vi "External Time to System Time.vi"(8 "error in (no error)":errorcluster, 9 "ClockID":u8, 10 "External Time":i64, 11 "Clock Convert Map in":T1) -> (0 "error out":errorcluster, 1 "Last Reset Time":u64, 2 "System Time":i64, 3 "Clock Convert Map out":T1)   [LabVIEW 2021, in "CIFClocks.lvlib"]
uses:
  CIFClocks.lvlib
  Typedef/Clock Conversion Map.ctl
  Typedef/Timestamp Pair.ctl
  CIFCore/Common/Typedef/Errors.ctl
  CIFCore/Common/Utilities/Append Error Location.vi
  CIFCore/Common/CIFCoreCommon.lvlib
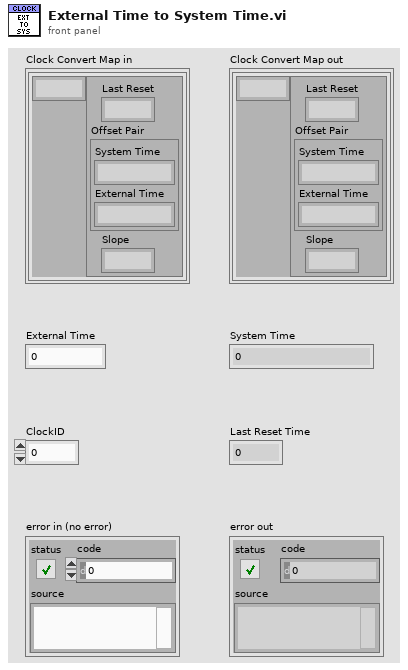
[diagram p1: front panel]
types:
  T1 = typedef "CIFClocks.lvlib/Clock Conversion Map.ctl" = map{u8, cluster{"Last Reset":u64, "Offset Pair":T2, "Slope":dbl}}
  T2 = typedef "CIFClocks.lvlib/Timestamp Pair.ctl" = cluster{"System Time":i64, "External Time":i64}
  T3 = cluster{"Last Reset":u64, "Offset Pair":T2, "Slope":dbl}
  T4 = typedef "CIFCoreCommon.lvlib/Errors.ctl" = enum16{"Invalid Clock ID", "Long Sleep", "gRPC Server Not Found", "Config Parse", "Timestamp Wrap", "Delayed Execution", "Duplicate Channel", "Missing Channel", "Incorrect Type", "Flatten Error", "Unflatten Data", "Unique Name", "Plugin Not Found", "Plugin Type Not Found", "Plugin Version Not Found", "Manager Not Found", "Numerical Issue", "Time Jump", "Clock ID Match", "Channel Length", "Plugin Connection", "gRPC Server Connection"}
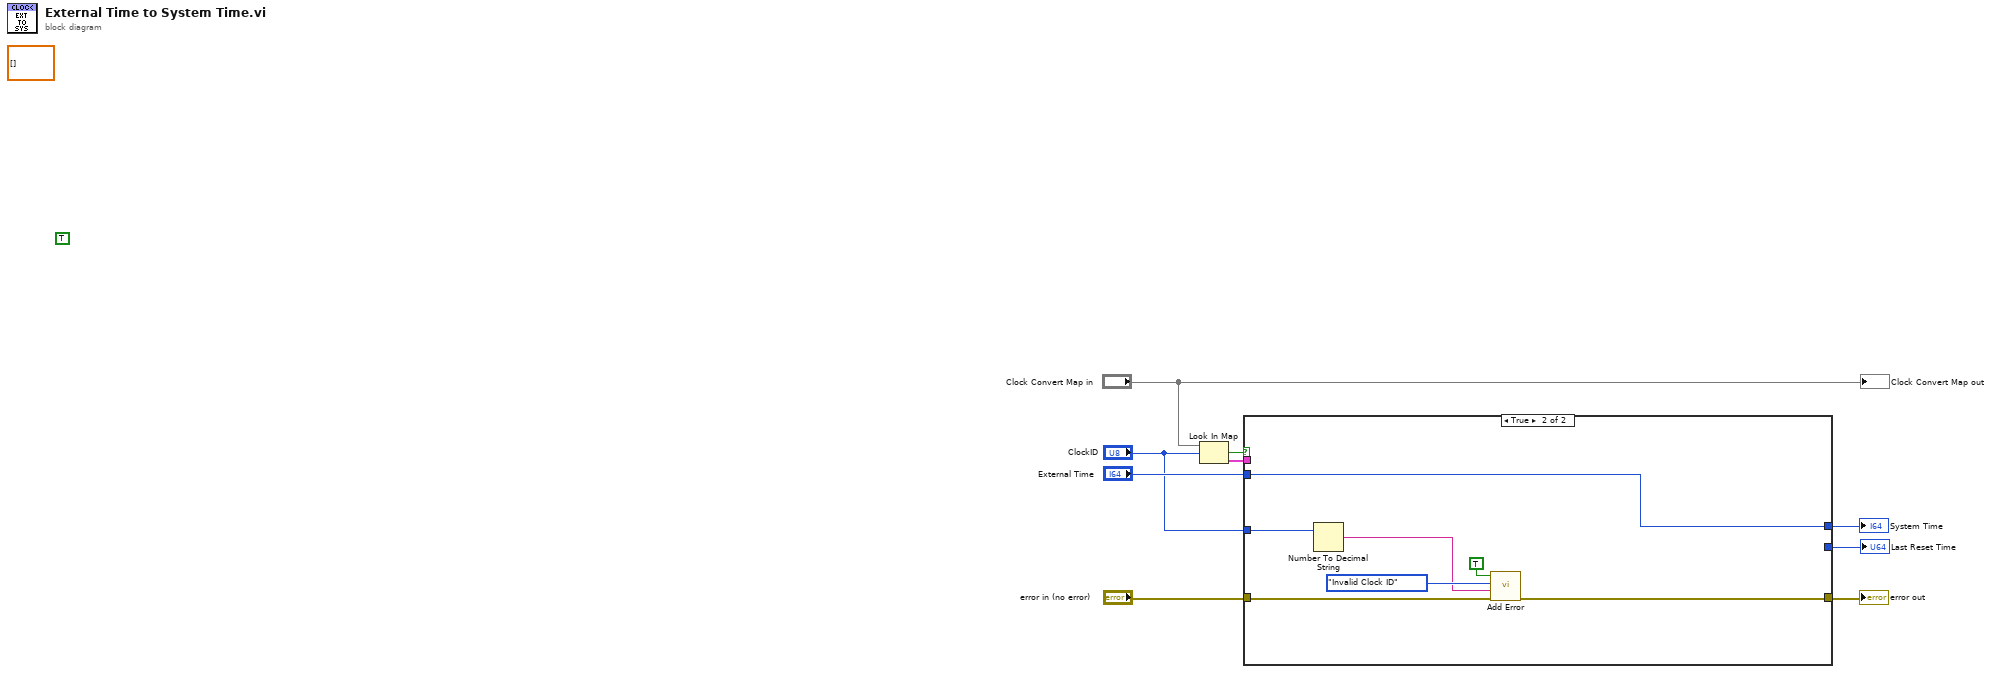
[diagram p0: block diagram]
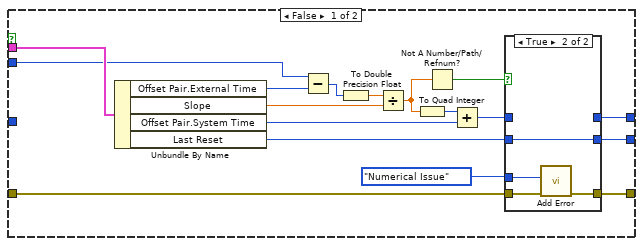
[diagram p2: hidden frame]
diagram:
  (unwired) TRUE
  (unwired) dbl[][] []
  n1 = Look In Map(map="Clock Convert Map in", key="ClockID") -> (key not found?=w4:bool, value=w9:T3)  [unwired: 1 in]
  n2 = case shown="True" w4 {
    tunnel: w9 -> [w26 _]
    tunnel: "External Time" -> [w19 w34]
    tunnel: [w13 w34] -> w7
    tunnel: [w14 _] -> w6
    tunnel: "error in (no error)" -> [w10 w37]
    tunnel: [w11 w36] -> w2
    tunnel: "ClockID" -> [_ w35]
    frame False {
      n3 = Unbundle By Name(w26) -> ("Offset Pair.External Time"=w21:i64, "Slope"=w25:dbl, "Offset Pair.System Time"=w20:i64, "Last Reset"=w15:u64)
      n4 = Subtract(x=w19, y=w21) -> (x-y=w24:i64)
      n5 = To Double Precision Float(number=w24) -> (double precision float=w23:dbl)
      n6 = Divide(x=w23, y=w25) -> (x/y=w18:dbl)
      n7 = To Quad Integer(1:w18) -> (0:w22:i64)
      n8 = Not A Number/Path/Refnum?(number/path/refnum=w18) -> (NaN/Path/Refnum?=w17:bool)
      n9 = Add(x=w22, y=w20) -> (x+y=w16:i64)
      n10 = case shown="True" w17 {
        tunnel: w16 -> [w28 _]
        tunnel: w15 -> [w29 w33]
        tunnel: [w29 w33] -> w14
        tunnel: [w28 _] -> w13
        tunnel: Errors."Numerical Issue" ("Error") -> [_ w32]
        tunnel: [w27 w31] -> w11
        tunnel: w10 -> [w27 w30]
        frame False {
        }
        frame True {
          n11 = call "Add Error.vi"("error in (no error)"=w30, "Error"=w32) -> ("error out"=w31:errorcluster)  [unwired: 9 in]
        }
      }
    }
    frame True {
      n12 = Number To Decimal String(number=w35) -> (decimal integer string=w38:string)  [unwired: 1 in]
      n13 = call "Add Error.vi"("error in (no error)"=w37, "String to Append"=w38, "Error"=Errors."Invalid Clock ID", "Insert Error"=TRUE) -> ("error out"=w36:errorcluster)  [unwired: 7 in]
    }
  }
  "System Time" <- w7
  "error out" <- w2
  "Last Reset Time" <- w6
  "Clock Convert Map out" <- "Clock Convert Map in"
